vi "reshape image data.vi"() -> ()   [LabVIEW 2015]
uses:
  LiveImage_Global.vi
  NIDAQControls/NIDAQGlobals.vi
panel:
  in  "Laser Mode":string
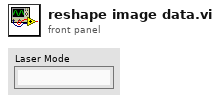
[diagram p1: front panel]
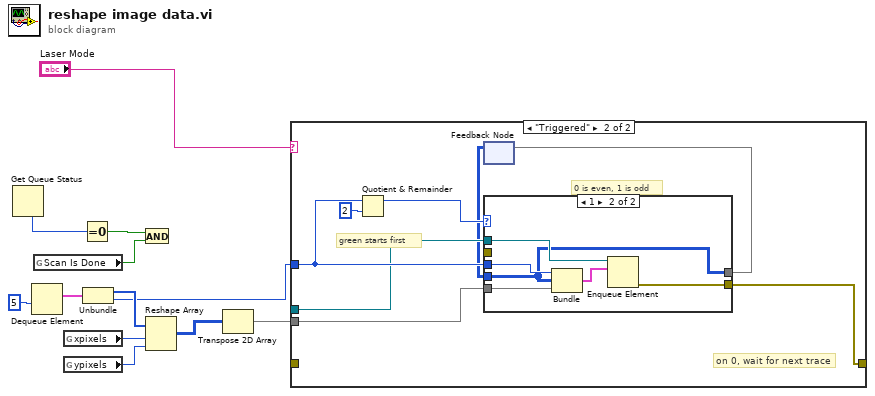
[diagram p0: block diagram]
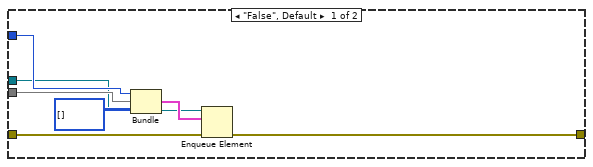
[diagram p2: hidden frame]
diagram:
  n1 = Get Queue Status() -> (# elements in queue=w8:i32)  [unwired: 3 in, 7 out]
  n2 = Dequeue Element(timeout in ms (-1)=5) -> (element=w11:cluster{u16[], i32})  [unwired: 2 in, 3 out]
  n3 = global read "NIDAQGlobals.vi" "Scan Is Done"() -> (w6:bool)
  n4 = global read "LiveImage_Global.vi" "xpixels"() -> (w13:i32)
  n5 = global read "LiveImage_Global.vi" "ypixels"() -> (w12:i32)
  n6 = Equal To 0?(x=w8) -> (x = 0?=w7:bool)
  n7 = Unbundle(w11) -> (w10:u16[], w4:i32)
  n8 = And(x=w7, y=w6) -> (x .and. y?=w5:bool)
  n9 = Reshape Array(w10, w13, w12) -> (w15:u16[][])
  n10 = Transpose 2D Array(2D array=w15) -> (transposed array=w14:u16[][])
  n11 = case shown="\"Triggered\"" "Laser Mode" {
    tunnel: w14 -> [w21 w28]
    tunnel: w4 -> [w19 w27]
    tunnel: [w16 w26] -> w3
    tunnel: _ -> [w18 _]
    tunnel: [w17 w23] -> w2
    frame "False", Default {
      n12 = Bundle(w19, w21, u16[][] []) -> (w22:cluster{i32, u16[][], u16[][]})  [unwired: 1 in]
      n13 = Enqueue Element(queue=w16, element=w22, error in (no error)=w18) -> (error out=w17:errorcluster)  [unwired: 1 in, 2 out]
    }
    frame "Triggered" {
      # "on 0, wait for next trace"
      # "0 is even, 1 is odd"
      # "green starts first"
      n14 = Quotient & Remainder(x=w27, y=2) -> (x-y*floor(x/y)=w29:i32)  [unwired: 1 out]
      n15 = feedback #1() -> (w24:u16[][])  [unwired: 1 in]
      n16 = case shown="1" w29 {
        tunnel: w28 -> [w32 w38]
        tunnel: w24 -> [_ w34]
        tunnel: w27 -> [_ w37]
        tunnel: w26 -> [_ w35]
        tunnel: [w32 w34] -> w25
        tunnel: _ -> [w31 _]
        tunnel: [w31 w33] -> w23
        frame 0, Default {
        }
        frame 1 {
          n17 = Bundle(w37, w34, w38) -> (w36:cluster{i32, u16[][], u16[][]})  [unwired: 1 in]
          n18 = Enqueue Element(queue=w35, element=w36) -> (error out=w33:errorcluster)  [unwired: 2 in, 2 out]
        }
      }
      n19 = feedback-in #1(w25) -> ()
    }
  }
